vi "getStatus.vi"(8 "error in (no error)":errorcluster, 10 "Status Name in":string, 11 "IComponent in":refnum<class "IComponentStatusContainer.lvclass">) -> (0 "error out":errorcluster, 2 "Status out":string, 3 "IComponent out":refnum<class "IComponentStatusContainer.lvclass">)   [LabVIEW 2022 SP3, in "openDAQ.lvlib" / "IBaseObject.lvlib" / "IComponentStatusContainer.lvlib" / "IComponentStatusContainer.lvclass"]
uses:
  <instrlib>/openDAQ/Public/Classes/IComponentStatusContainer/IComponentStatusContainer.lvclass
  C:/Program Files (x86)/National Instruments/LabVIEW 2022/instr.lib/openDAQ/Public/Classes/IBaseObject/IBaseObject.lvclass
  <instrlib>/openDAQ/Public/Classes/daqCoreTypes/IEnumeration/IEnumeration.lvclass
  <instrlib>/openDAQ/Public/Classes/IBaseObject/IBaseObject.lvclass/IBaseObject.ctl
  <instrlib>/openDAQ/Public/Classes/IBaseObject/Accessor/Read reference.vi
  <instrlib>/openDAQ/Public/Classes/IBaseObject/Accessor/Write reference.vi
  <instrlib>/openDAQ/Public/Classes/daqCoreTypes/IString/IString.lvclass
  <instrlib>/openDAQ/Binaries/Windows/x86/copendaq32.dll
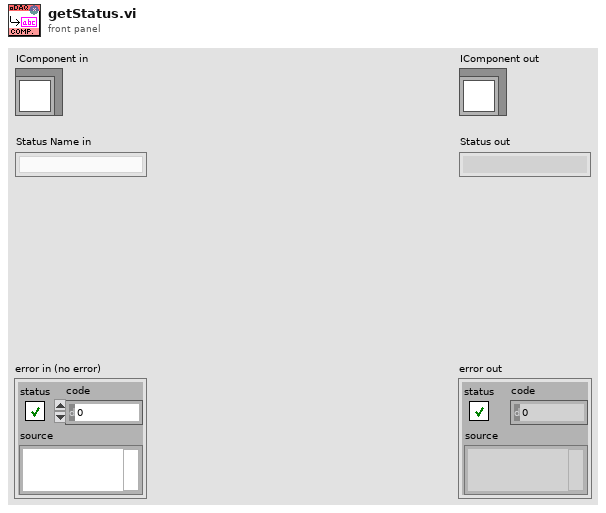
[diagram p1: front panel]
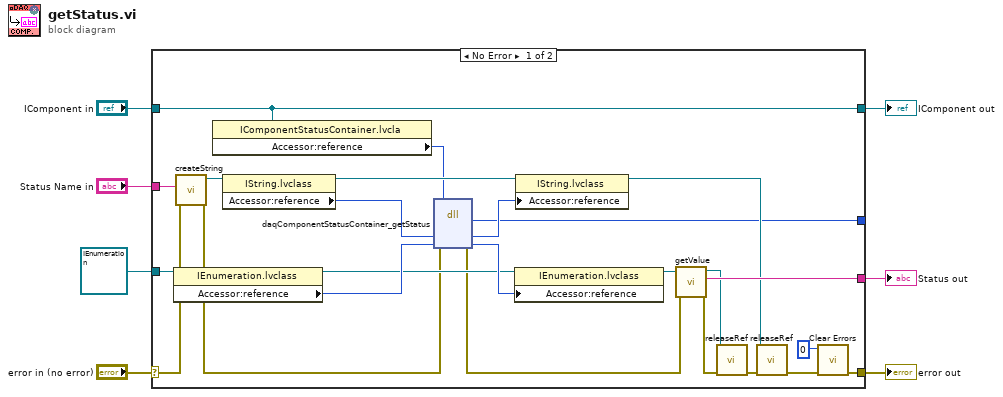
[diagram p0: block diagram]
diagram:
  n1 = case shown="No Error" "error in (no error)" {
    selector: "error in (no error)" -> [w23 w33]
    tunnel: [w10 w33] -> w6
    tunnel: [w9 w32] -> w4
    tunnel: "IComponent in" -> [w9 w32]
    tunnel: refnum<class "IEnumeration.lvclass"> refnum ("openDAQ.lvlib:daqCoreTypes.lvlib:IEnumeration.lvclass") -> [w27 _]
    tunnel: [w25 _] -> w3
    tunnel: "Status Name in" -> [w21 _]
    tunnel: [w15 _] -> _
    frame No Error {
      n2 = property class="IEnumeration.lvclass"(reference=w27) -> (reference out=w29:refnum<class "IEnumeration.lvclass">, "Accessor:reference"=w31:i64)  [unwired: 1 in, 1 out]
      n3 = call <instrlib>:"createString.vi"("error in (no error)"=w23, "String"=w21) -> ("error out"=w22:errorcluster, "IString out"=w20:refnum<class "IString.lvclass">)  [unwired: 8 in]
      n4 = property class="IComponentStatusContainer.lvcla"(reference=w9) -> ("Accessor:reference"=w8:i64)  [unwired: 1 in, 2 out]
      n5 = property class="IString.lvclass"(reference=w20) -> (reference out=w18:refnum<class "IString.lvclass">, "Accessor:reference"=w19:i64)  [unwired: 1 in, 1 out]
      n6 = dll-call lib="C:/Program Files (x86)/National Instruments/LabVIEW 2022/instr.lib/openDAQ/Binaries/Windows/x86/copendaq*.*" fn="daqComponentStatusContainer_getStatus"(error in=w22, "device"=w8, "name"=w19, "value"=w31) -> (error out=w14:errorcluster, "err"=w15:u32, "name"=w28:i64, "value"=w30:i64)  [unwired: 3 in, 1 out]
      n7 = property class="IEnumeration.lvclass"(reference=w29, "Accessor:reference"=w30) -> (reference out=w26:refnum<class "IEnumeration.lvclass">)  [unwired: 1 in, 1 out]
      n8 = property class="IString.lvclass"(reference=w18, "Accessor:reference"=w28) -> (reference out=w16:refnum<class "IString.lvclass">)  [unwired: 1 in, 1 out]
      n9 = call <instrlib>:"getValue.vi"("error in (no error)"=w14, "Enumeration in"=w26) -> ("error out"=w13:errorcluster, "Value out"=w25:string, "Enumeration out"=w24:refnum<class "IEnumeration.lvclass">)  [unwired: 7 in]
      n10 = call-dynamic "releaseRef.vi"("error in (no error)"=w13, "IBaseObject in"=w24) -> ("error out"=w17:errorcluster)  [unwired: 9 in]
      n11 = call-dynamic "releaseRef.vi"("error in (no error)"=w17, "IBaseObject in"=w16) -> ("error out"=w11:errorcluster)  [unwired: 9 in]
      n12 = call <vilib>:"Clear Errors.vi"("error in (no error)"=w11, "specific error code to clear (0: all)"=0) -> ("error out"=w10:errorcluster)  [unwired: 4 in, 1 out]
    }
    frame Error {
    }
  }
  "error out" <- w6
  "IComponent out" <- w4
  "Status out" <- w3
